vi "Delete_Element.vi"(2 "error in (no error)":errorcluster, 3 "Numeric":i32, 4 "Queue in":refnum<queue>) -> (0 "error out":errorcluster, 1 "Queue out":refnum<queue>)   [LabVIEW 2018]
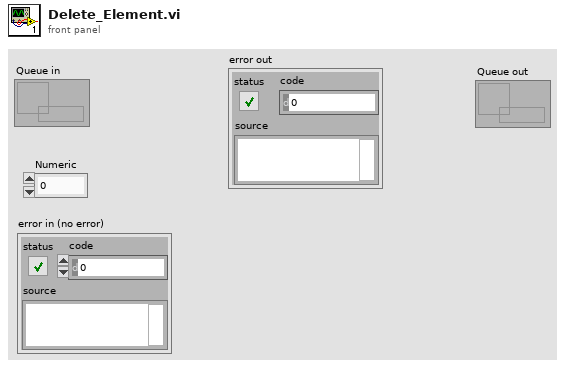
[diagram p1: front panel]
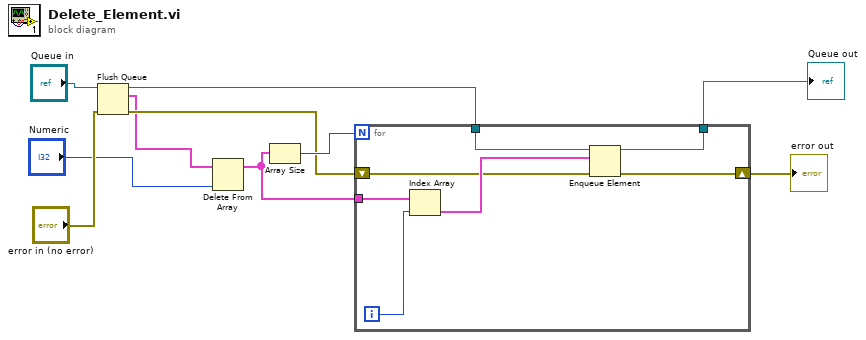
[diagram p0: block diagram]
diagram:
  n1 = Flush Queue(queue="Queue in", error in (no error)="error in (no error)") -> (queue out=w8:refnum<queue>, remaining elements=w3:cluster{"Test Name":string, "File Path":path}[], error out=w4:errorcluster)
  n2 = Delete From Array(array=w3, index="Numeric") -> (array with subset deleted=w1:cluster{"Test Name":string, "File Path":path}[])  [unwired: 1 in, 1 out]
  n3 = Array Size(array=w1) -> (size(s)=w9:i32)
  n4 = for {
    N: w9 -> [_]
    tunnel: w8 -> [w17]
    tunnel: w1 -> [w16]
    tunnel: [w13] -> w6
    shift-right: [w12] -> w5
    shift-left: w4 -> [w11]
    i -> [w15]
    n5 = Index Array(array=w16, index=w15) -> (element=w14:cluster{"Test Name":string, "File Path":path})
    n6 = Enqueue Element(queue=w17, element=w14, error in (no error)=w11) -> (queue out=w13:refnum<queue>, error out=w12:errorcluster)  [unwired: 1 in, 1 out]
  }
  "Queue out" <- w6
  "error out" <- w5
